vi "VisionPnPPose.vi"(8 "Previous Y Estimate (in)":dbl, 9 "LimeLight Raw X (in)":dbl, 10 "LimeLight Raw Z (in)":dbl, 11 "Previous X Estimate (in)":dbl) -> (1 "deltaY (in)":dbl, 2 "deltaX (in)":dbl)   [LabVIEW 2019]
doc: "This VI converts the raw LimeLight pipeline values into the global field coordinate system."
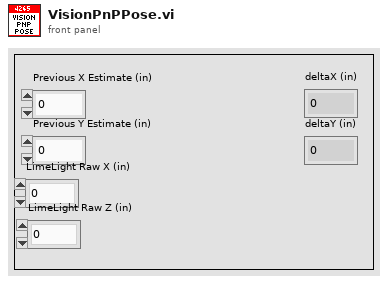
[diagram p1: front panel]
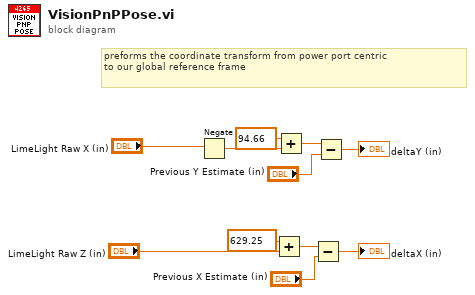
[diagram p0: block diagram]
diagram:
  # "preforms the coordinate transform from power port centric\nto our global reference frame"
  n1 = Negate(x="LimeLight Raw X (in)") -> (-x=w11:dbl)
  n2 = Add(x=629.25, y="LimeLight Raw Z (in)") -> (x+y=w7:dbl)
  n3 = Add(x=94.66, y=w11) -> (x+y=w10:dbl)
  n4 = Subtract(x=w7, y="Previous X Estimate (in)") -> (x-y=→"deltaX (in)":dbl)
  n5 = Subtract(x=w10, y="Previous Y Estimate (in)") -> (x-y=→"deltaY (in)":dbl)
